vi "화12조.vi"() -> ()   [LabVIEW 2020]
uses:
  <vilib>/DAQmx/read.llb/DAQmx Read (Digital Bool 1Line 1Point).vi
  <vilib>/DAQmx/write.llb/DAQmx Write (Analog 1D Wfm NChan NSamp).vi
  <vilib>/DAQmx/miscellaneous.llb/DAQmx Fill In Error Info.vi
panel:
  in  "정지":bool
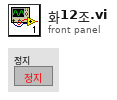
[diagram p1: front panel]
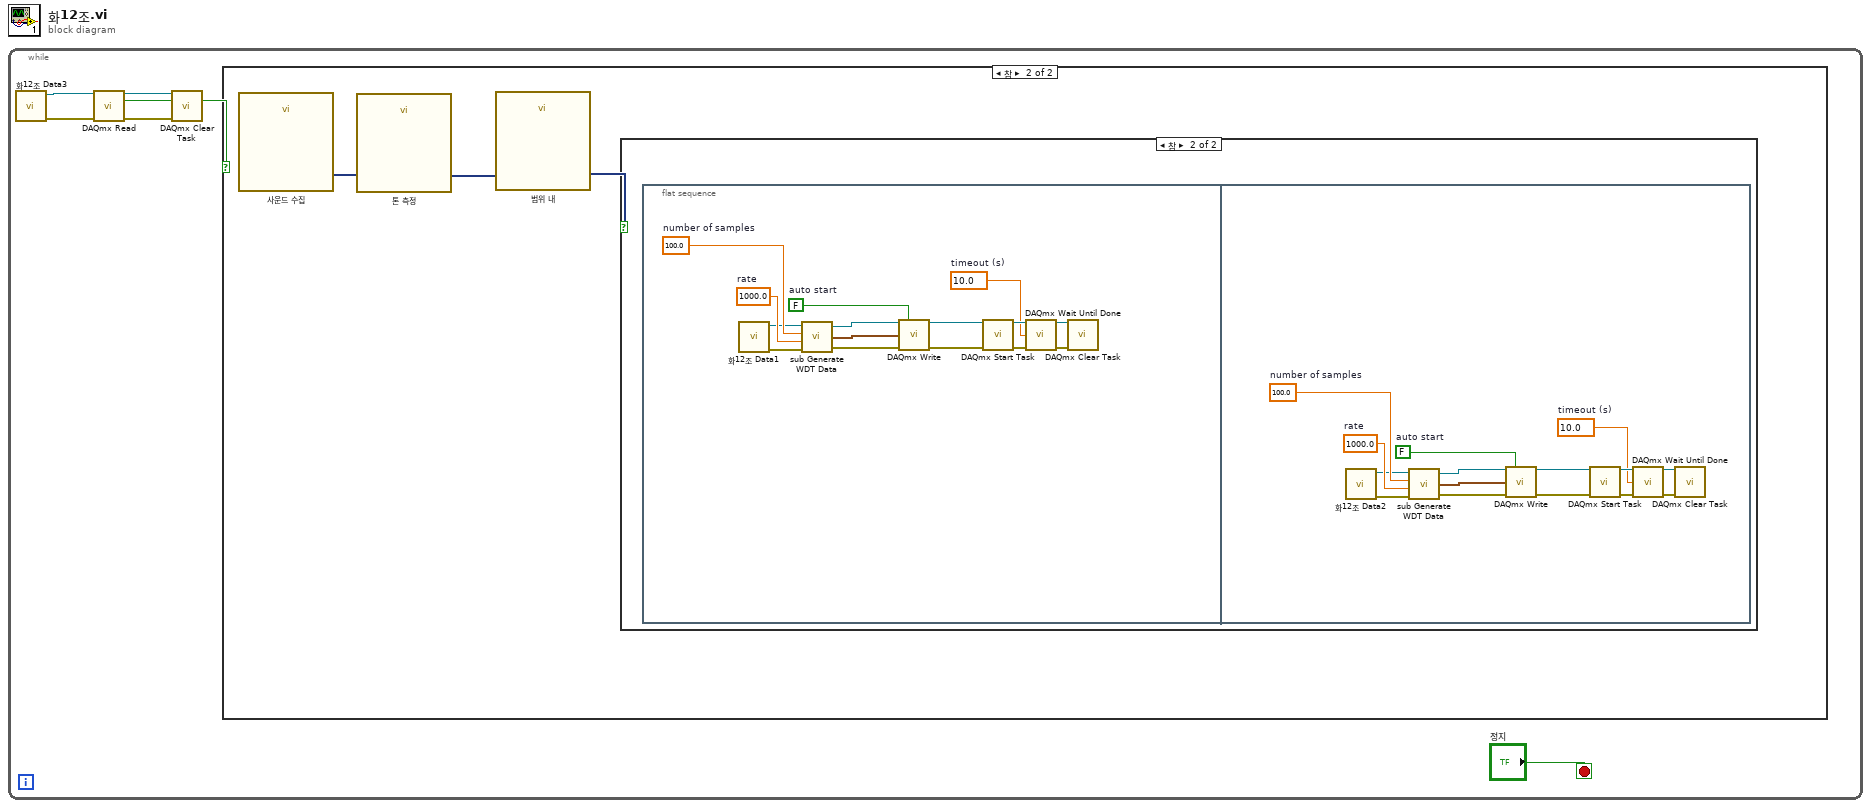
[diagram p0: block diagram]
diagram:
  n1 = while {
    stop <- "정지" stop-if-true
    n2 = call "화12조 Data3.vi"() -> ("error out"=w5:errorcluster, "task out"=w4:refnum<k21>)  [unwired: 10 in]
    n3 = call-poly <vilib>:"DAQmx Read.vi"("task/channels in"=w4, "error in"=w5) -> ("task out"=w3:refnum<k21>, "data"=w1:bool, "error out"=w2:errorcluster)  [unwired: 11 in]
    n4 = call <vilib>:"DAQmx Clear Task.vi"("task in"=w3, "error in"=w2) -> ()  [unwired: 13 in, 1 out]
    n5 = case shown="참" w1 {
      frame False {
      }
      frame True {
        n6 = call "사운드 수집"() -> ("Data"=w9:dynamicdata)  [unwired: 18 in, 1 out]
        n7 = call "톤 측정"("Signals"=w9) -> ("Frequency"=w8:dynamicdata)  [unwired: 9 in, 1 out]
        n8 = call "범위 내"("Operand 1"=w8) -> ("Result"=w7:dynamicdata)  [unwired: 9 in, 1 out]
        n9 = case shown="참" w7 {
          frame False {
          }
          frame True {
            n10 = flat-sequence {
              frame #0 {
                w15 = 10.0  # timeout (s)
                w19 = 1000.0  # rate
                w20 = 100.0  # number of samples
                w24 = FALSE  # auto start
                n11 = call "화12조 Data1.vi"() -> ("error out"=w10:errorcluster, "task out"=w11:refnum<k21>)  [unwired: 10 in]
                n12 = call <vilib>:"sub Generate WDT Data.vi"("task in"=w11, "number of samples"=w20, "update rate"=w19, "error in"=w10) -> ("task out"=w22:refnum<k21>, "Data"=w21:waveform(dbl)[], "error out"=w23:errorcluster)  [unwired: 1 in]
                n13 = call-poly <vilib>:"DAQmx Write.vi"("task/channels in"=w22, "auto start"=w24, "data"=w21, "error in"=w23) -> ("task out"=w14:refnum<k21>, "error out"=w13:errorcluster)  [unwired: 9 in, 1 out]
                n14 = call <vilib>:"DAQmx Start Task.vi"("task/channels in"=w14, "error in"=w13) -> ("task out"=w18:refnum<k21>, "error out"=w17:errorcluster)  [unwired: 12 in]
                n15 = call <vilib>:"DAQmx Wait Until Done.vi"("task/channels in"=w18, "timeout (sec)"=w15, "error in"=w17) -> ("task out"=w12:refnum<k21>, "error out"=w16:errorcluster)  [unwired: 11 in]
                n16 = call <vilib>:"DAQmx Clear Task.vi"("task in"=w12, "error in"=w16) -> ()  [unwired: 13 in, 1 out]
              }
              frame #1 {
                w30 = 10.0  # timeout (s)
                w34 = 1000.0  # rate
                w35 = 100.0  # number of samples
                w39 = FALSE  # auto start
                n17 = call "화12조 Data2.vi"() -> ("error out"=w25:errorcluster, "task out"=w26:refnum<k21>)  [unwired: 10 in]
                n18 = call <vilib>:"sub Generate WDT Data.vi"("task in"=w26, "number of samples"=w35, "update rate"=w34, "error in"=w25) -> ("task out"=w37:refnum<k21>, "Data"=w36:waveform(dbl)[], "error out"=w38:errorcluster)  [unwired: 1 in]
                n19 = call-poly <vilib>:"DAQmx Write.vi"("task/channels in"=w37, "auto start"=w39, "data"=w36, "error in"=w38) -> ("task out"=w29:refnum<k21>, "error out"=w28:errorcluster)  [unwired: 9 in, 1 out]
                n20 = call <vilib>:"DAQmx Start Task.vi"("task/channels in"=w29, "error in"=w28) -> ("task out"=w33:refnum<k21>, "error out"=w32:errorcluster)  [unwired: 12 in]
                n21 = call <vilib>:"DAQmx Wait Until Done.vi"("task/channels in"=w33, "timeout (sec)"=w30, "error in"=w32) -> ("task out"=w27:refnum<k21>, "error out"=w31:errorcluster)  [unwired: 11 in]
                n22 = call <vilib>:"DAQmx Clear Task.vi"("task in"=w27, "error in"=w31) -> ()  [unwired: 13 in, 1 out]
              }
            }
          }
        }
      }
    }
  }
